vi "Waveform.vi"() -> ()   [LabVIEW 2018]
panel:
  out "Waveform Graph":dbl[](graph)
  out "Waveform Array":dbl[](array[numeric])
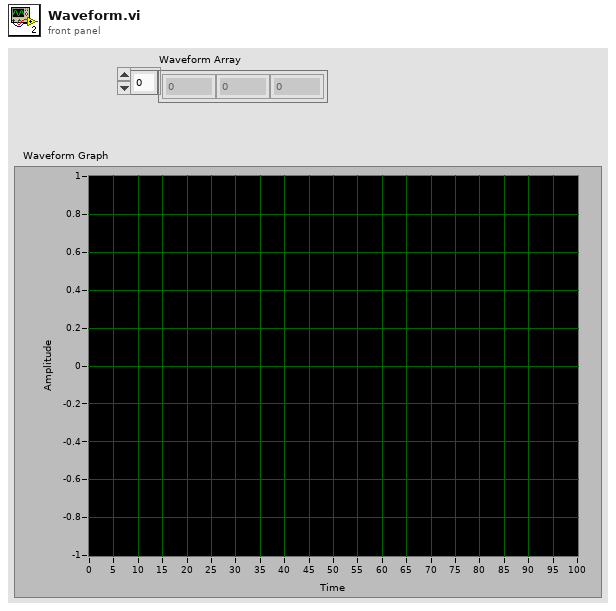
[diagram p1: front panel]
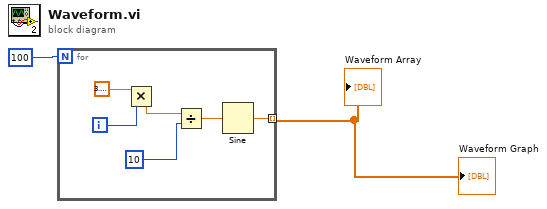
[diagram p0: block diagram]
diagram:
  n1 = for {
    N: 100 -> [_]
    tunnel: [w4] -> w1 mode=indexing
    i -> [w3]
    n2 = Multiply(x=3.141592653589793, y=w3) -> (x*y=w6:dbl)
    n3 = Divide(x=w6, y=10) -> (x/y=w8:dbl)
    n4 = Sine(x=w8) -> (sin(x)=w4:dbl)
  }
  "Waveform Array" <- w1
  "Waveform Graph" <- w1
